vi "testONR.vi"() -> ()   [LabVIEW 2011]
panel:
  in  "Boolean":bool
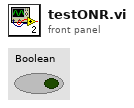
[diagram p1: front panel]
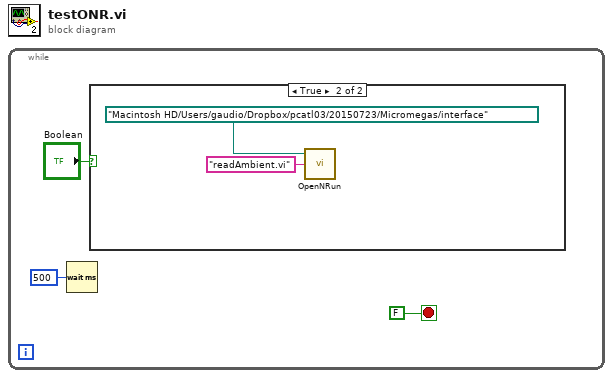
[diagram p0: block diagram]
diagram:
  n1 = while {
    stop <- FALSE stop-if-true
    n2 = Wait (ms)(milliseconds to wait=u32 500) -> ()  [unwired: 1 out]
    n3 = case shown="True" "Boolean" {
      frame False {
      }
      frame True {
        n4 = call "OpenNRun.vi"("VI name"="readAmbient.vi", "ViDirPath"=path "/Macintosh HD/Users/gaudio/Dropbox/pcatl03/20150723/Micromegas/interface") -> ()  [unwired: 1 in]
      }
    }
  }
